vi "getText.vi"(0 "reference":refnum<class "MultiLineString.lvclass">, 5 "error in (no error)":errorcluster) -> (14 "reference out":refnum<class "MultiLineString.lvclass">, 15 "text":string, 19 "error out":errorcluster)   [LabVIEW 2014, in "MultiLineString.lvclass"]
doc: "public String getText()"
uses:
  <resource>/Framework/Providers/Open_GDS/UML/MultiLineString_class/MultiLineString.lvclass
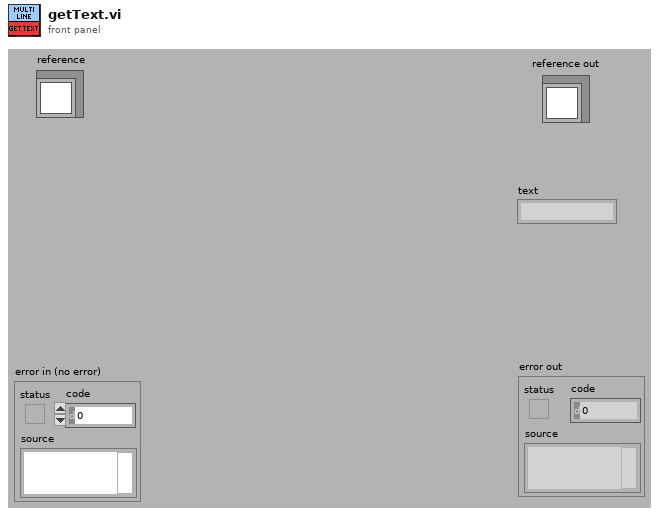
[diagram p1: front panel]
types:
  T1 = typedef "MultiLineString.lvclass/ObjectAttributes.ctl" = cluster{"GAP":i32, "text":string, "justification":T2, "size":T3, "underlined":bool}
  T2 = typedef "MultiLineString.lvclass/JustificationType.ctl" = enum16{"LEFT", "CENTER", "RIGHT"}
  T3 = typedef "MultiLineString.lvclass/SizeType.ctl" = enum16{"LARGE", "NORMAL", "SMALL"}
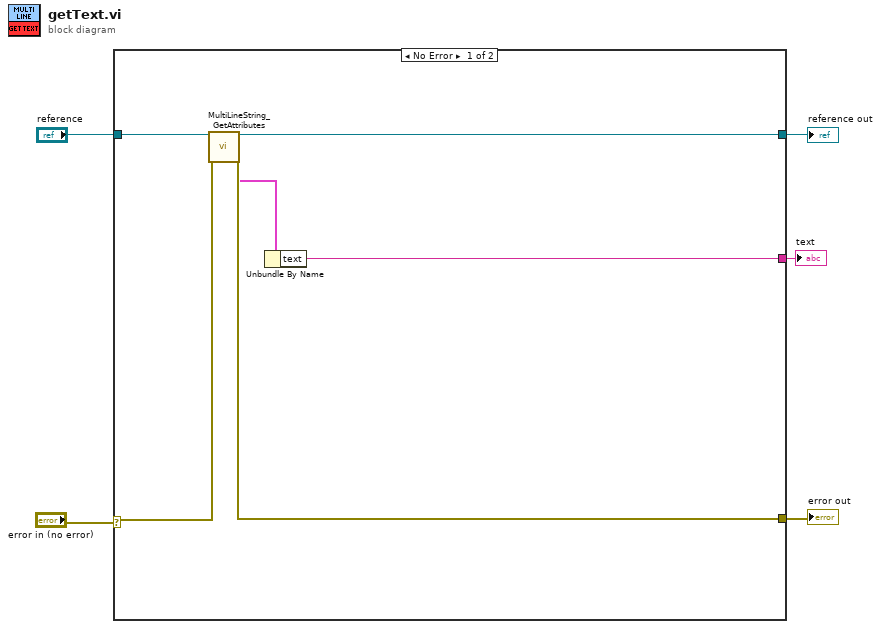
[diagram p0: block diagram]
diagram:
  n1 = case shown="No Error" "error in (no error)" {
    selector: "error in (no error)" -> [w8 w12]
    tunnel: "reference" -> [w11 w13]
    tunnel: [w10 w12] -> w3
    tunnel: [w9 w13] -> w2
    tunnel: [w7 _] -> w1
    frame No Error {
      n2 = call <resource>:"MultiLineString_GetAttributes.vi"("reference in"=w11, "error in (no error)"=w8) -> ("reference out"=w9:refnum<class "MultiLineString.lvclass">, "Data"=w6:T1, "error out"=w10:errorcluster)  [unwired: 1 in, 14 out]
      n3 = Unbundle By Name(w6) -> ("text"=w7:string)
    }
    frame Error {
    }
  }
  "reference out" <- w2
  "error out" <- w3
  "text" <- w1
